vi "Read Keys Refnum.vi"(8 "error in (no error)":errorcluster, 11 "Configuration UI in":refnum<class "Configuration UI.lvclass">) -> (0 "error out":errorcluster, 2 "Keys Refnum":refnum<vi>, 3 "Configuration UI out":refnum<class "Configuration UI.lvclass">)   [LabVIEW 2019, in "Configuration UI.lvlib" / "Configuration UI.lvclass"]
uses:
  Project/Configuration UI.lvclass
  Project/Configuration UI.lvclass/Configuration UI.ctl
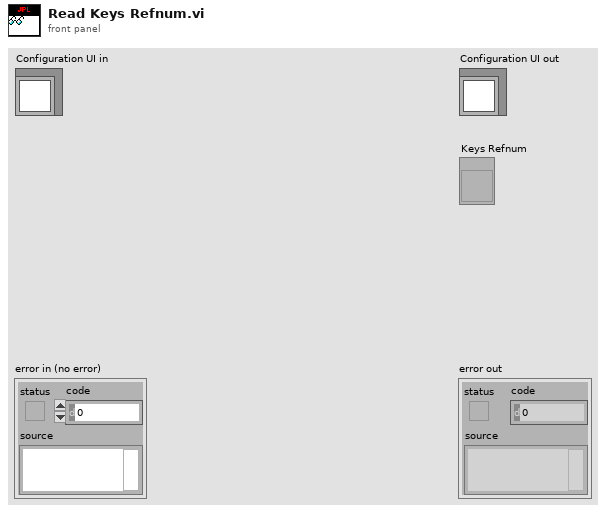
[diagram p1: front panel]
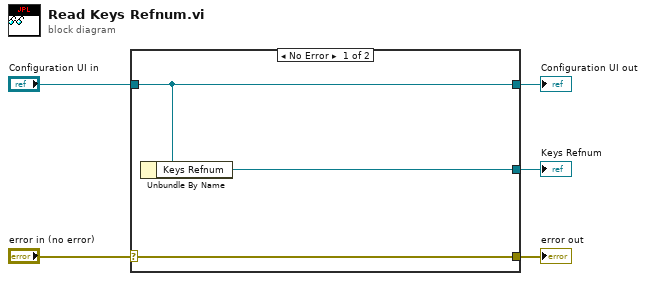
[diagram p0: block diagram]
diagram:
  n1 = case shown="No Error" "error in (no error)" {
    selector: "error in (no error)" -> [w8 w9]
    tunnel: [w8 w9] -> w4
    tunnel: [w7 w10] -> w2
    tunnel: "Configuration UI in" -> [w7 w10]
    tunnel: [w6 _] -> w1
    frame No Error {
      n2 = Unbundle By Name(w7) -> ("Keys Refnum"=w6:refnum<vi>)
    }
    frame Error {
    }
  }
  "error out" <- w4
  "Configuration UI out" <- w2
  "Keys Refnum" <- w1
